vi "Sony LANC remote.vi"() -> ()   [LabVIEW 2023]
panel:
  in  "plus":bool
  in  "minus":bool
  in  "15key":bool
  in  "16key":bool
  in  "7key":bool
  in  "8key":bool
  in  "9key":bool
  in  "10key":bool
  in  "11key":bool
  in  "12key":bool
  in  "13key":bool
  in  "14key":bool
  in  "1key":bool caption="Keypad"
  in  "2key":bool
  in  "3key":bool
  in  "4key":bool
  in  "5key":bool
  in  "6key":bool
  in  "EEPROM_store":bool
  in  "EEPROM_read":bool
  in  "valup":bool caption="Data"
  in  "valdn":bool
  in  "adup":bool caption="Addr"
  in  "addn":bool
  in  "pgup":bool caption="Page"
  in  "pgdn":bool
  out "EEPROM":string
  in  "send_custom":bool
  in  "eject":bool
  in  "fwd":bool
  in  "rew":bool
  in  "stop":bool
  in  "pause":bool
  in  "play":bool
  in  "enter":bool
  in  "menu":bool
  in  "right":bool
  in  "left":bool
  in  "up":bool
  in  "down":bool
  in  "Command":string(combo)
  out "Time":string
  out "Date":string
  out "data_code":cluster{"year/hour":u32, "month/min":u32}
  out "data_type":u8(ring) items=["Undefined"=0, "Date"=3, "Time"=4]
  out "Remaining time":string
  out "Real time counter":string
  out "RCTC":bool
  out "min_sec":cluster{"min":u32, "sec":u32}
  out "Decimal counter":u32
  out "Features":T1 {"Capability" items=["V8"=0, "DV"=1, "DV"=2, "Hi8"=4]; "Input" items=["Tuner"=0, "Sim."=1, "Line"=3]; "Thickness" items=["10µm", "13µm"]; "Type" items=["MP", "ME"]; "Speed" items=["SP", "LP"]}
  out "Status":string
  out "EOP":bool
  in  "stop":bool
  in  "send":bool
  in  "cmd":string caption="Custom cmd (2 bytes hex)"
  # "Tape"
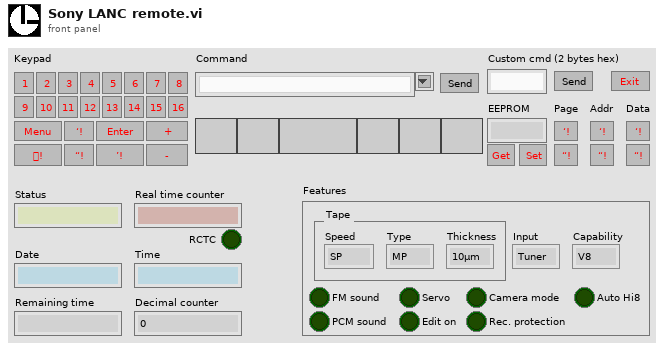
[diagram p1: front panel]
types:
  T1 = cluster{"Speed":u8, "FM sound":bool, "PCM sound":bool, "Camera mode":bool, "Rec. protection":bool, "Type":u8, "Thickness":u8, "Servo":bool, "Input":u8, "Capability":u8, "Edit on":bool, "Auto Hi8":bool}
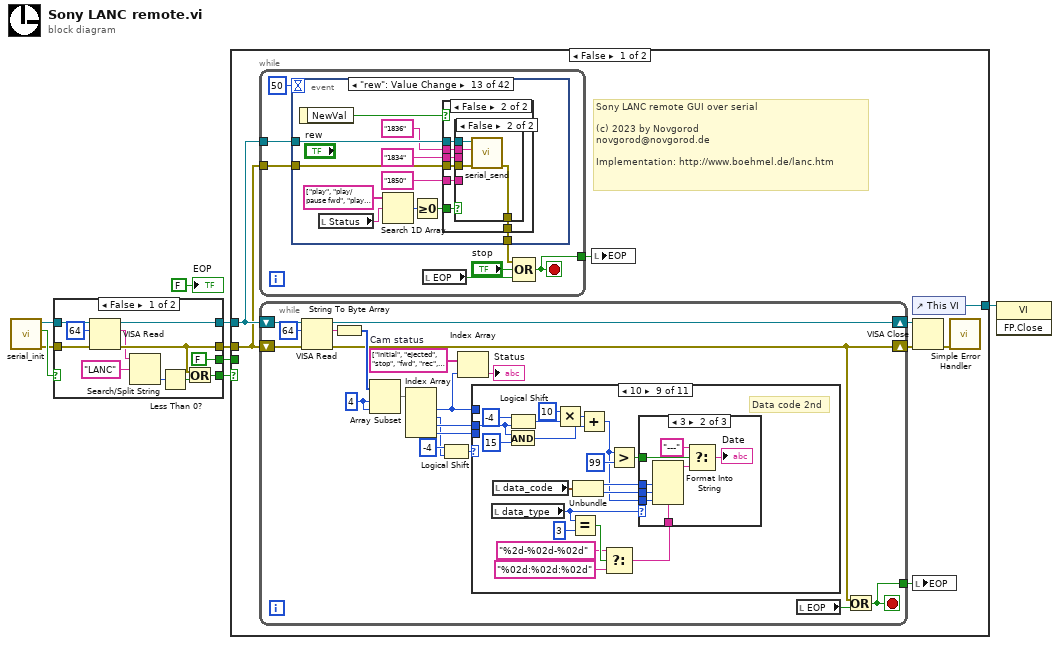
[diagram p0: block diagram]
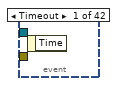
[diagram p3: hidden frame]
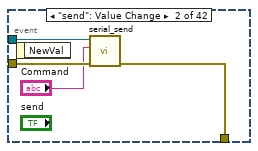
[diagram p4: hidden frame]
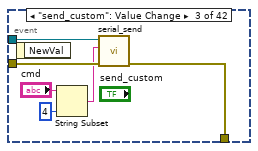
[diagram p5: hidden frame]
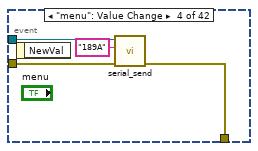
[diagram p6: hidden frame]
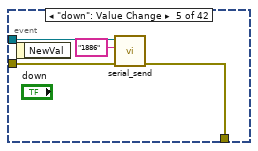
[diagram p7: hidden frame]
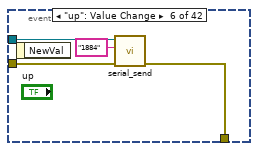
[diagram p8: hidden frame]
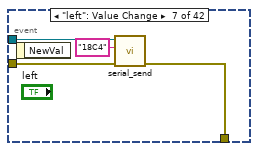
[diagram p9: hidden frame]
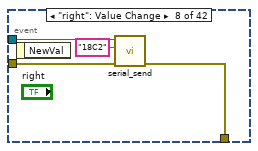
[diagram p10: hidden frame]
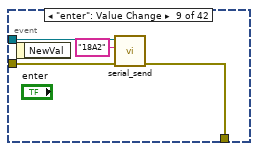
[diagram p11: hidden frame]
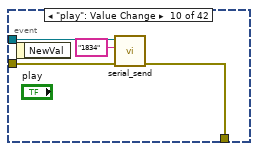
[diagram p12: hidden frame]
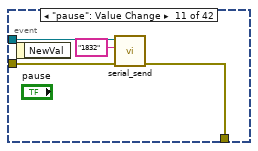
[diagram p13: hidden frame]
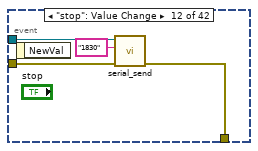
[diagram p14: hidden frame]
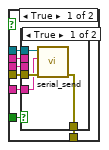
[diagram p15: hidden frame]
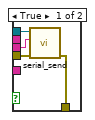
[diagram p17: hidden frame]
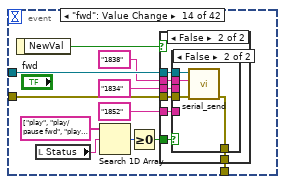
[diagram p18: hidden frame]
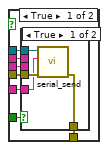
[diagram p19: hidden frame]
diagram:
  n1 = call "serial_init.vi"() -> ("error out"=w3:errorcluster, "Cancelled?"=w4:bool, "VISA out"=w5:refnum<visa-resource-name>)  [unwired: 9 in]
  n2 = case shown="False" w4 {
    selector: w4 -> [_ w21]
    tunnel: [w20 w22] -> w9
    tunnel: [w19 _] -> w8
    tunnel: [w18 w21] -> w7
    tunnel: w5 -> [w12 w22]
    tunnel: w3 -> [w11 _]
    tunnel: [FALSE w21] -> w1
    frame False {
      n3 = VISA Read(VISA resource name=w12, byte count=u32 64, error in (no error)=w11) -> (VISA resource name out=w20:refnum<visa-resource-name>, read buffer=w16:string, error out=w19:errorcluster)  [unwired: 1 out]
      n4 = Search/Split String(string=w16, search string/char (-)="LANC") -> (offset of match=w14:i32)  [unwired: 1 in, 2 out]
      n5 = Less Than 0?(x=w14) -> (x < 0?=w13:bool)
      n6 = Or(x=w19, y=w13) -> (x .or. y?=w18:bool)
    }
    frame True {
    }
  }
  n7 = case shown="False" w7 {
    tunnel: w9 -> [w27 w470]
    tunnel: w8 -> [w26 _]
    tunnel: [w23 w471] -> w2
    tunnel: w1 -> [_ w469]
    frame False {
      # "Sony LANC remote GUI over serial\n\n(c) 2023 by Novgorod\nnovgorod@novgorod.de\n\nImplementation: http://www.boehmel.de/lanc.htm"
      n8 = while {
        tunnel: w26 -> [w35]
        tunnel: w27 -> [w36]
        tunnel: [w32] -> w24
        stop <- w32 stop-if-true
        n9 = event shown="[12] \"rew\": Value Change" {
          selector: _ -> [_ _ _ _ _ _ _ _ _ _ _ _ _ _ _ _ _ _ _ _ _ _ _ _ _ _ _ _ _ _ _ _ _ _ _ _ _ _ _ _ _ _]
          dyn-events: _ -> [_ _ _ _ _ _ _ _ _ _ _ _ _ _ _ _ _ _ _ _ _ _ _ _ _ _ _ _ _ _ _ _ _ _ _ _ _ _ _ _ _ _]
          timeout: 50 -> [_ _ _ _ _ _ _ _ _ _ _ _ _ _ _ _ _ _ _ _ _ _ _ _ _ _ _ _ _ _ _ _ _ _ _ _ _ _ _ _ _ _]
          tunnel: w36 -> [_ w41 w47 w51 w55 w59 w63 w67 w71 w75 w79 w83 w94 w132 w163 w167 w171 w175 w179 w183 w187 w191 w195 w199 w203 w207 w211 w215 w219 w223 w227 w231 w236 w245 w249 w253 w257 w261 w265 w269 w273 _]
          tunnel: w35 -> [_ w40 w46 w50 w54 w58 w62 w66 w70 w74 w78 w82 w93 w131 w162 w166 w170 w174 w178 w182 w186 w190 w194 w198 w202 w206 w210 w214 w218 w222 w226 w230 w235 w244 w248 w252 w256 w260 w264 w268 w272 _]
          tunnel: [_ w39 w45 w49 w53 w57 w61 w65 w69 w73 w77 w81 w92 w130 w161 w165 w169 w173 w177 w181 w185 w189 w193 w197 w201 w205 w209 w213 w217 w221 w225 w229 w234 w243 w247 w251 w255 w259 w263 w267 w271 errorcluster {"status"=TRUE, "code"=0, "source"=""} ("error out")] -> w34
          event Timeout {
            n10 = event-data() -> ()  [unwired: 1 in, 1 out]
          }
          event "send": Value Change {
            n11 = event-data() -> ()  [unwired: 1 in, 1 out]
            n12 = call "serial_send.vi"("error in (no error)"=w40, "Send buffer"="Command", "VISA in"=w41) -> ("error out"=w39:errorcluster)  [unwired: 7 in, 1 out]
          }
          event "send_custom": Value Change {
            n13 = event-data() -> ()  [unwired: 1 in, 1 out]
            n14 = String Subset(string="cmd", length (rest)=4 ("length (rest)")) -> (substring=w42:string)  [unwired: 1 in]
            n15 = call "serial_send.vi"("error in (no error)"=w46, "Send buffer"=w42, "VISA in"=w47) -> ("error out"=w45:errorcluster)  [unwired: 7 in, 1 out]
          }
          event "menu": Value Change {
            n16 = event-data() -> ()  [unwired: 1 in, 1 out]
            n17 = call "serial_send.vi"("error in (no error)"=w50, "Send buffer"="189A", "VISA in"=w51) -> ("error out"=w49:errorcluster)  [unwired: 7 in, 1 out]
          }
          event "down": Value Change {
            n18 = event-data() -> ()  [unwired: 1 in, 1 out]
            n19 = call "serial_send.vi"("error in (no error)"=w54, "Send buffer"="1886", "VISA in"=w55) -> ("error out"=w53:errorcluster)  [unwired: 7 in, 1 out]
          }
          event "up": Value Change {
            n20 = event-data() -> ()  [unwired: 1 in, 1 out]
            n21 = call "serial_send.vi"("error in (no error)"=w58, "Send buffer"="1884", "VISA in"=w59) -> ("error out"=w57:errorcluster)  [unwired: 7 in, 1 out]
          }
          event "left": Value Change {
            n22 = event-data() -> ()  [unwired: 1 in, 1 out]
            n23 = call "serial_send.vi"("error in (no error)"=w62, "Send buffer"="18C4", "VISA in"=w63) -> ("error out"=w61:errorcluster)  [unwired: 7 in, 1 out]
          }
          event "right": Value Change {
            n24 = event-data() -> ()  [unwired: 1 in, 1 out]
            n25 = call "serial_send.vi"("error in (no error)"=w66, "Send buffer"="18C2", "VISA in"=w67) -> ("error out"=w65:errorcluster)  [unwired: 7 in, 1 out]
          }
          event "enter": Value Change {
            n26 = event-data() -> ()  [unwired: 1 in, 1 out]
            n27 = call "serial_send.vi"("error in (no error)"=w70, "Send buffer"="18A2", "VISA in"=w71) -> ("error out"=w69:errorcluster)  [unwired: 7 in, 1 out]
          }
          event "play": Value Change {
            n28 = event-data() -> ()  [unwired: 1 in, 1 out]
            n29 = call "serial_send.vi"("error in (no error)"=w74, "Send buffer"="1834", "VISA in"=w75) -> ("error out"=w73:errorcluster)  [unwired: 7 in, 1 out]
          }
          event "pause": Value Change {
            n30 = event-data() -> ()  [unwired: 1 in, 1 out]
            n31 = call "serial_send.vi"("error in (no error)"=w78, "Send buffer"="1832", "VISA in"=w79) -> ("error out"=w77:errorcluster)  [unwired: 7 in, 1 out]
          }
          event "stop": Value Change {
            n32 = event-data() -> ()  [unwired: 1 in, 1 out]
            n33 = call "serial_send.vi"("error in (no error)"=w82, "Send buffer"="1830", "VISA in"=w83) -> ("error out"=w81:errorcluster)  [unwired: 7 in, 1 out]
          }
          event "rew": Value Change {
            n34 = event-data() -> ("NewVal"=w87:bool)  [unwired: 1 in]
            n35 = local read "Status"() -> (w89:string)
            n36 = Search 1D Array(1D array=string[] ["play", "play/pause fwd", "play/pause rev", "cue", "rev", "x1 fwd", "1/5 fwd", "x1 rev", "1/5 rev", "1/10 fwd", "1/10 rev", "x2/x3 fwd", "x2/x3 rev", "x9 fwd", "x9 rev", "edit-s rev", "frame sea. rev", "x14 fwd", "x14 rev", "edit search+", "edit search-", "edit-s fwd", "frame sea. cue"], element=w89) -> (index of element=w90:i32)  [unwired: 1 in]
            n37 = Greater Or Equal To 0?(x=w90) -> (x >= 0?=w88:bool)
            n38 = case shown="False" w87 {
              tunnel: w94 -> [w101 w113]
              tunnel: w93 -> [w100 w112]
              tunnel: [w99 w111] -> w92
              tunnel: "1836" -> [w98 w110]
              tunnel: w88 -> [w97 w109]
              tunnel: "1850" -> [w96 w108]
              tunnel: "1834" -> [w95 w107]
              frame True {
                n39 = case shown="True" w97 {
                  tunnel: w101 -> [w105 _]
                  tunnel: w100 -> [w104 w106]
                  tunnel: [w103 w106] -> w99
                  tunnel: w98 -> [_ _]
                  tunnel: w96 -> [w102 _]
                  tunnel: w95 -> [_ _]
                  frame True {
                    n40 = call "serial_send.vi"("error in (no error)"=w104, "Send buffer"=w102, "VISA in"=w105) -> ("error out"=w103:errorcluster)  [unwired: 7 in, 1 out]
                  }
                  frame False {
                  }
                }
              }
              frame False {
                n41 = case shown="False" w109 {
                  tunnel: w113 -> [w117 w119]
                  tunnel: w112 -> [w116 w121]
                  tunnel: [w115 w118] -> w111
                  tunnel: w110 -> [_ w120]
                  tunnel: w108 -> [_ _]
                  tunnel: w107 -> [w114 _]
                  frame True {
                    n42 = call "serial_send.vi"("error in (no error)"=w116, "Send buffer"=w114, "VISA in"=w117) -> ("error out"=w115:errorcluster)  [unwired: 7 in, 1 out]
                  }
                  frame False {
                    n43 = call "serial_send.vi"("error in (no error)"=w121, "Send buffer"=w120, "VISA in"=w119) -> ("error out"=w118:errorcluster)  [unwired: 7 in, 1 out]
                  }
                }
              }
            }
          }
          event "fwd": Value Change {
            n44 = event-data() -> ("NewVal"=w125:bool)  [unwired: 1 in]
            n45 = local read "Status"() -> (w127:string)
            n46 = Search 1D Array(1D array=string[] ["play", "play/pause fwd", "play/pause rev", "cue", "rev", "x1 fwd", "1/5 fwd", "x1 rev", "1/5 rev", "1/10 fwd", "1/10 rev", "x2/x3 fwd", "x2/x3 rev", "x9 fwd", "x9 rev", "edit-s rev", "frame sea. rev", "x14 fwd", "x14 rev", "edit search+", "edit search-", "edit-s fwd", "frame sea. cue"], element=w127) -> (index of element=w128:i32)  [unwired: 1 in]
            n47 = Greater Or Equal To 0?(x=w128) -> (x >= 0?=w126:bool)
            n48 = case shown="False" w125 {
              tunnel: w132 -> [w139 w151]
              tunnel: w131 -> [w138 w150]
              tunnel: [w137 w149] -> w130
              tunnel: "1838" -> [w136 w148]
              tunnel: w126 -> [w135 w147]
              tunnel: "1852" -> [w134 w146]
              tunnel: "1834" -> [w133 w145]
              frame True {
                n49 = case shown="True" w135 {
                  tunnel: w139 -> [w143 _]
                  tunnel: w138 -> [w142 w144]
                  tunnel: [w141 w144] -> w137
                  tunnel: w136 -> [_ _]
                  tunnel: w134 -> [w140 _]
                  tunnel: w133 -> [_ _]
                  frame True {
                    n50 = call "serial_send.vi"("error in (no error)"=w142, "Send buffer"=w140, "VISA in"=w143) -> ("error out"=w141:errorcluster)  [unwired: 7 in, 1 out]
                  }
                  frame False {
                  }
                }
              }
              frame False {
                n51 = case shown="False" w147 {
                  tunnel: w151 -> [w155 w158]
                  tunnel: w150 -> [w154 w159]
                  tunnel: [w153 w156] -> w149
                  tunnel: w148 -> [_ w157]
                  tunnel: w146 -> [_ _]
                  tunnel: w145 -> [w152 _]
                  frame True {
                    n52 = call "serial_send.vi"("error in (no error)"=w154, "Send buffer"=w152, "VISA in"=w155) -> ("error out"=w153:errorcluster)  [unwired: 7 in, 1 out]
                  }
                  frame False {
                    n53 = call "serial_send.vi"("error in (no error)"=w159, "Send buffer"=w157, "VISA in"=w158) -> ("error out"=w156:errorcluster)  [unwired: 7 in, 1 out]
                  }
                }
              }
            }
          }
          event "1key": Value Change {
            n54 = event-data() -> ()  [unwired: 1 in, 1 out]
            n55 = call "serial_send.vi"("error in (no error)"=w162, "Send buffer"="1800", "VISA in"=w163) -> ("error out"=w161:errorcluster)  [unwired: 7 in, 1 out]
          }
          event "2key": Value Change {
            n56 = event-data() -> ()  [unwired: 1 in, 1 out]
            n57 = call "serial_send.vi"("error in (no error)"=w166, "Send buffer"="1802", "VISA in"=w167) -> ("error out"=w165:errorcluster)  [unwired: 7 in, 1 out]
          }
          event "3key": Value Change {
            n58 = event-data() -> ()  [unwired: 1 in, 1 out]
            n59 = call "serial_send.vi"("error in (no error)"=w170, "Send buffer"="1804", "VISA in"=w171) -> ("error out"=w169:errorcluster)  [unwired: 7 in, 1 out]
          }
          event "4key": Value Change {
            n60 = event-data() -> ()  [unwired: 1 in, 1 out]
            n61 = call "serial_send.vi"("error in (no error)"=w174, "Send buffer"="1806", "VISA in"=w175) -> ("error out"=w173:errorcluster)  [unwired: 7 in, 1 out]
          }
          event "5key": Value Change {
            n62 = event-data() -> ()  [unwired: 1 in, 1 out]
            n63 = call "serial_send.vi"("error in (no error)"=w178, "Send buffer"="1808", "VISA in"=w179) -> ("error out"=w177:errorcluster)  [unwired: 7 in, 1 out]
          }
          event "6key": Value Change {
            n64 = event-data() -> ()  [unwired: 1 in, 1 out]
            n65 = call "serial_send.vi"("error in (no error)"=w182, "Send buffer"="180A", "VISA in"=w183) -> ("error out"=w181:errorcluster)  [unwired: 7 in, 1 out]
          }
          event "7key": Value Change {
            n66 = event-data() -> ()  [unwired: 1 in, 1 out]
            n67 = call "serial_send.vi"("error in (no error)"=w186, "Send buffer"="180C", "VISA in"=w187) -> ("error out"=w185:errorcluster)  [unwired: 7 in, 1 out]
          }
          event "8key": Value Change {
            n68 = event-data() -> ()  [unwired: 1 in, 1 out]
            n69 = call "serial_send.vi"("error in (no error)"=w190, "Send buffer"="180E", "VISA in"=w191) -> ("error out"=w189:errorcluster)  [unwired: 7 in, 1 out]
          }
          event "9key": Value Change {
            n70 = event-data() -> ()  [unwired: 1 in, 1 out]
            n71 = call "serial_send.vi"("error in (no error)"=w194, "Send buffer"="1810", "VISA in"=w195) -> ("error out"=w193:errorcluster)  [unwired: 7 in, 1 out]
          }
          event "10key": Value Change {
            n72 = event-data() -> ()  [unwired: 1 in, 1 out]
            n73 = call "serial_send.vi"("error in (no error)"=w198, "Send buffer"="1812", "VISA in"=w199) -> ("error out"=w197:errorcluster)  [unwired: 7 in, 1 out]
          }
          event "11key": Value Change {
            n74 = event-data() -> ()  [unwired: 1 in, 1 out]
            n75 = call "serial_send.vi"("error in (no error)"=w202, "Send buffer"="1814", "VISA in"=w203) -> ("error out"=w201:errorcluster)  [unwired: 7 in, 1 out]
          }
          event "12key": Value Change {
            n76 = event-data() -> ()  [unwired: 1 in, 1 out]
            n77 = call "serial_send.vi"("error in (no error)"=w206, "Send buffer"="1816", "VISA in"=w207) -> ("error out"=w205:errorcluster)  [unwired: 7 in, 1 out]
          }
          event "13key": Value Change {
            n78 = event-data() -> ()  [unwired: 1 in, 1 out]
            n79 = call "serial_send.vi"("error in (no error)"=w210, "Send buffer"="1818", "VISA in"=w211) -> ("error out"=w209:errorcluster)  [unwired: 7 in, 1 out]
          }
          event "14key": Value Change {
            n80 = event-data() -> ()  [unwired: 1 in, 1 out]
            n81 = call "serial_send.vi"("error in (no error)"=w214, "Send buffer"="181A", "VISA in"=w215) -> ("error out"=w213:errorcluster)  [unwired: 7 in, 1 out]
          }
          event "15key": Value Change {
            n82 = event-data() -> ()  [unwired: 1 in, 1 out]
            n83 = call "serial_send.vi"("error in (no error)"=w218, "Send buffer"="181C", "VISA in"=w219) -> ("error out"=w217:errorcluster)  [unwired: 7 in, 1 out]
          }
          event "16key": Value Change {
            n84 = event-data() -> ()  [unwired: 1 in, 1 out]
            n85 = call "serial_send.vi"("error in (no error)"=w222, "Send buffer"="181E", "VISA in"=w223) -> ("error out"=w221:errorcluster)  [unwired: 7 in, 1 out]
          }
          event "plus": Value Change {
            n86 = event-data() -> ()  [unwired: 1 in, 1 out]
            n87 = call "serial_send.vi"("error in (no error)"=w226, "Send buffer"="1820", "VISA in"=w227) -> ("error out"=w225:errorcluster)  [unwired: 7 in, 1 out]
          }
          event "minus": Value Change {
            n88 = event-data() -> ()  [unwired: 1 in, 1 out]
            n89 = call "serial_send.vi"("error in (no error)"=w230, "Send buffer"="1822", "VISA in"=w231) -> ("error out"=w229:errorcluster)  [unwired: 7 in, 1 out]
          }
          event "eject": Value Change {
            n90 = event-data() -> ()  [unwired: 1 in, 1 out]
            n91 = Two Button Dialog(message="Eject tape?") -> (T button?=w232:bool)  [unwired: 2 in]
            n92 = case shown="True" w232 {
              tunnel: w236 -> [_ w241]
              tunnel: w235 -> [w237 w240]
              tunnel: [w237 w239] -> w234
              frame False {
              }
              frame True {
                n93 = call "serial_send.vi"("error in (no error)"=w240, "Send buffer"="182C", "VISA in"=w241) -> ("error out"=w239:errorcluster)  [unwired: 7 in, 1 out]
              }
            }
          }
          event "EEPROM_read": Value Change {
            n94 = event-data() -> ()  [unwired: 1 in, 1 out]
            n95 = call "serial_send.vi"("error in (no error)"=w244, "Send buffer"="FF00", "VISA in"=w245) -> ("error out"=w243:errorcluster)  [unwired: 7 in, 1 out]
          }
          event "EEPROM_store": Value Change {
            n96 = event-data() -> ()  [unwired: 1 in, 1 out]
            n97 = call "serial_send.vi"("error in (no error)"=w248, "Send buffer"="FF32", "VISA in"=w249) -> ("error out"=w247:errorcluster)  [unwired: 7 in, 1 out]
          }
          event "pgup": Value Change {
            n98 = event-data() -> ()  [unwired: 1 in, 1 out]
            n99 = call "serial_send.vi"("error in (no error)"=w252, "Send buffer"="FF67", "VISA in"=w253) -> ("error out"=w251:errorcluster)  [unwired: 7 in, 1 out]
          }
          event "pgdn": Value Change {
            n100 = event-data() -> ()  [unwired: 1 in, 1 out]
            n101 = call "serial_send.vi"("error in (no error)"=w256, "Send buffer"="FF65", "VISA in"=w257) -> ("error out"=w255:errorcluster)  [unwired: 7 in, 1 out]
          }
          event "adup": Value Change {
            n102 = event-data() -> ()  [unwired: 1 in, 1 out]
            n103 = call "serial_send.vi"("error in (no error)"=w260, "Send buffer"="FF38", "VISA in"=w261) -> ("error out"=w259:errorcluster)  [unwired: 7 in, 1 out]
          }
          event "addn": Value Change {
            n104 = event-data() -> ()  [unwired: 1 in, 1 out]
            n105 = call "serial_send.vi"("error in (no error)"=w264, "Send buffer"="FF36", "VISA in"=w265) -> ("error out"=w263:errorcluster)  [unwired: 7 in, 1 out]
          }
          event "valup": Value Change {
            n106 = event-data() -> ()  [unwired: 1 in, 1 out]
            n107 = call "serial_send.vi"("error in (no error)"=w268, "Send buffer"="FF34", "VISA in"=w269) -> ("error out"=w267:errorcluster)  [unwired: 7 in, 1 out]
          }
          event "valdn": Value Change {
            n108 = event-data() -> ()  [unwired: 1 in, 1 out]
            n109 = call "serial_send.vi"("error in (no error)"=w272, "Send buffer"="FF30", "VISA in"=w273) -> ("error out"=w271:errorcluster)  [unwired: 7 in, 1 out]
          }
          event Panel Close? {
            n110 = event-data() -> ()  [unwired: 1 in, 1 out]
            n111 = event-data("Discard?"=TRUE) -> ()  [unwired: 1 in, 1 out]
          }
        }
        n112 = local read "EOP"() -> (w31:bool)
        n113 = Compound Arithmetic op=OR(w34, "stop", w31) -> (w32:bool)
      }
      n114 = while {
        shift-right: [w292] -> w29
        shift-left: w27 -> [w294]
        shift-right: [w287] -> w30
        shift-left: w26 -> [w293]
        tunnel: [w276] -> w25
        stop <- w276 stop-if-true
        w284 = string[] ["initial", "ejected", "stop", "fwd", "rec", "", "play", "play/pause fwd", "AL insert", "", "", "", "", "", "", "page 0", "", "dew cass. out", "laod", "", "rec/pause", "", "", "frame fwd", "AL ins-pause", "", "", "", "", "", "", "page 1", "", "ejecting", "cassette busy", "", "timer-rec", "", "x1 fwd", "1/5 fwd", "AR insert", "", "", "", "", "", "", "page 2", "", "unload", "low-battery", "go zero/play f.", "timer-rec s.", "", "x1 rev", "1/5 rev", "AR ins-pause", "", "", "", "", "", "", "page 3", "", "", "dew stop", "fwd mem stop", "AV insert", "", "cue", "1/10 fwd", "AL+V insert", "", "", "", "", "", "", "page 4", "", "", "emergency", "", "AV ins.-pause", "", "rev", "1/10 rev", "AL+V ins-ps", "", "", "", "", "", "", "page 5", "", "", "tape end", "", "video insert", "", "x2/x3 fwd", "frame fwd", "AR+V insert", "", "", "", "", "", "", "page 6", "", "", "tape top", "", "video ins.-ps", "", "x2/x3 rev", "frame rev", "AL+R ins-ps", "", "", "", "", "", "", "page 7", "", "", "", "rew", "audio dub", "edit search+", "x9 fwd", "", "", "", "", "", "", "", "", "page 8", "", "", "stp after zero", "", "a. dub pause", "edit search-", "x9 rev", "play/pause rev", "", "", "", "", "", "", "", "page 9", "", "", "load emer.", "auto-play", "cam rec", "edit-s fwd", "frame sea. cue", "", "", "", "", "", "", "", "", "page A", "", "unload emerg.", "stop emerg. 1", "go zero/play r.", "cam stby", "edit-s rev", "frame sea. rev", "", "", "", "", "", "", "", "", "page B", "", "", "stop emerg. 2", "rew mem stop", "", "", "x14 fwd", "", "", "", "", "", "", "", "", "page C", "", "", "", "hi-speed rew", "", "", "x14 rev", "", "", "", "", "", "", "", "", "page D", "", "", "stop NC", "", "", "", "", "", "", "", "", "", "", "", "", "page E", "", "", "", "", "", "edit pause", "", "", "", "", "", "", "", "", "", "page F"]  # Cam status
        w286 = 4 ("index")
        n115 = VISA Read(VISA resource name=w294, byte count=u32 64, error in (no error)=w293) -> (VISA resource name out=w292:refnum<visa-resource-name>, read buffer=w290:string, error out=w287:errorcluster)  [unwired: 1 out]
        n116 = String To Byte Array(string=w290) -> (unsigned byte array=w289:u8[])
        n117 = Array Subset(array=w289, index=w286, length=w286) -> (w285:u8[])
        n118 = Index Array(array=w285) -> (element #1=w277:u8, element #2=w278:u8, element #3=w279:u8, element #4=w280:u8)  [unwired: 4 in]
        n119 = Logical Shift(y=i16 -4, x=w278) -> (x << y=w281:u8)
        n120 = Index Array(array=w284, index=w277) -> (element=→"Status":string)
        n121 = case shown="10" w281 {
          tunnel: w280 -> [_ w317 w330 w347 w374 w396 w399 w411 _ w456 w463]
          tunnel: w279 -> [_ w318 w331 w348 w382 w397 _ w412 w433 w460 w464]
          tunnel: w277 -> [_ _ _ _ _ _ _ _ _ _ w468]
          frame 0, Default {
          }
          frame 1 {
            # "Status V8 and Hi8"
            n122 = Join Numbers(hi=w317, lo=w318) -> ((hi.lo)=w316:u16)
            n123 = Number To Boolean Array(number=w316) -> (Boolean array=w315:bool[])
            n124 = Index Array(array=w315, index #2=2 ("index"), index #8=11 ("index"), index #10=14 ("index")) -> (element #1=w314:bool, element #2=w303:bool, element #3=w302:bool, element #4=w301:bool, element #5=w300:bool, element #6=w312:bool, element #7=w311:bool, element #8=w297:bool, element #9=w309:bool, element #10=w307:bool)  [unwired: 7 in]
            n125 = Boolean To (0,1)(Boolean=w314) -> (0, 1=w304:i16)
            n126 = Boolean To (0,1)(Boolean=w312) -> (0, 1=w299:i16)
            n127 = Boolean To (0,1)(Boolean=w311) -> (0, 1=w298:i16)
            n128 = Build Array(w309, w307) -> (w306:bool[])
            n129 = local read "Features"() -> (w305:T1)
            n130 = Boolean Array To Number(Boolean array=w306) -> (number=w296:u32)
            n131 = Bundle(cluster=w305, "Speed"=w304, "FM sound"=w303, "PCM sound"=w302, "Camera mode"=w301, "Rec. protection"=w300, "Type"=w299, "Thickness"=w298, "Servo"=w297, "Input"=w296) -> (→"Features":T1)  [unwired: 3 in]
          }
          frame 2 {
            # "Decimal counter"
            n132 = Logical Shift(y=i16 -4, x=w330) -> (x << y=w326:u8)
            n133 = And(x=w330, y=u8 15) -> (x .and. y?=w324:u8)
            n134 = Logical Shift(y=i16 -4, x=w331) -> (x << y=w329:u8)
            n135 = And(x=w331, y=u8 15) -> (x .and. y?=w322:u8)
            n136 = Multiply(x=u32 10, y=w329) -> (x*y=w323:u32)
            n137 = Multiply(x=u32 1000, y=w326) -> (x*y=w321:u32)
            n138 = Multiply(x=u32 100, y=w324) -> (x*y=w320:u32)
            n139 = Compound Arithmetic op=ADD(w323, w322, w321, w320) -> (→"Decimal counter":u32)
          }
          frame 3 {
            # "Real time counter 1st"
            n140 = Logical Shift(y=i16 -4, x=w347) -> (x << y=w343:u8)
            n141 = And(x=w347, y=u8 15) -> (x .and. y?=w339:u8)
            n142 = Logical Shift(y=i16 -4, x=w348) -> (x << y=w346:u8)
            n143 = And(x=w348, y=u8 15) -> (x .and. y?=w341:u8)
            n144 = Multiply(x=u32 10, y=w346) -> (x*y=w342:u32)
            n145 = Multiply(x=u32 10, y=w343) -> (x*y=w340:u32)
            n146 = Add(x=w342, y=w341) -> (x+y=w337:u32)
            n147 = Add(x=w340, y=w339) -> (x+y=w338:u32)
            n148 = Bundle(w338, w337) -> (→"min_sec":cluster{u32, u32})  [unwired: 1 in]
          }
          frame 4 {
            # "Real time counter 2nd"
            n149 = Number To Boolean Array(number=w374) -> (Boolean array=w373:bool[])
            n150 = Logical Shift(y=i16 -4, x=w374) -> (x << y=w361:u8)
            n151 = And(x=w374, y=u8 15) -> (x .and. y?=w375:u8)
            n152 = Logical Shift(y=i16 -4, x=w382) -> (x << y=w381:u8)
            n153 = And(x=w382, y=u8 15) -> (x .and. y?=w377:u8)
            n154 = Index Array(array=w373, index #1=6 ("index")) -> (element #1=→"RCTC":bool, element #2=w370:bool)  [unwired: 1 in]
            n155 = local read "min_sec"() -> (w364:cluster{"min":u32, "sec":u32})
            n156 = And(x=u8 3, y=w361) -> (x .and. y?=w359:u8)
            n157 = Multiply(x=u32 10, y=w381) -> (x*y=w378:u32)
            n158 = Add(x=w378, y=w377) -> (x+y=w358:u32)
            n159 = Multiply(x=u32 10, y=w359) -> (x*y=w376:u32)
            n160 = Select(t="-", s=w370, f="") -> (s? t:f=w367:string)
            n161 = Unbundle(w364) -> ("min"=w363:u32, "sec"=w362:u32)
            n162 = Add(x=w376, y=w375) -> (x+y=w365:u32)
            n163 = Greater?(x=w358, y=u32 99) -> (0:w356:bool)
            n164 = Format Into String(format string="%d:%02d:%02d:%02d", initial string=w367, w358, w363, w362, w365) -> (resulting string=w355:string)  [unwired: 1 in, 1 out]
            n165 = Select(t="---", s=w356, f=w355) -> (s? t:f=→"Real time counter":string)
          }
          frame 5 {
            w388 = u8 15
            # "Remaining time"
            n166 = Logical Shift(y=i16 -4, x=w397) -> (x << y=w395:u8)
            n167 = And(x=w397, y=w388) -> (x .and. y?=w392:u8)
            n168 = And(x=w396, y=w388) -> (x .and. y?=w389:u8)
            n169 = Multiply(x=u32 10, y=w395) -> (x*y=w393:u32)
            n170 = Add(x=w393, y=w392) -> (x+y=w390:u32)
            n171 = Format Into String(format string="%d:%02d", w389, w390) -> (resulting string=→"Remaining time":string)  [unwired: 2 in, 1 out]
          }
          frame 8 {
            # "Data code type"
            "data_type" <- w399
          }
          frame 9 {
            # "Data code 1st"
            n172 = Logical Shift(y=i16 -4, x=w411) -> (x << y=w407:u8)
            n173 = And(x=w411, y=u8 15) -> (x .and. y?=w403:u8)
            n174 = Logical Shift(y=i16 -4, x=w412) -> (x << y=w410:u8)
            n175 = And(x=w412, y=u8 15) -> (x .and. y?=w405:u8)
            n176 = Multiply(x=u32 10, y=w410) -> (x*y=w406:u32)
            n177 = Multiply(x=u32 10, y=w407) -> (x*y=w404:u32)
            n178 = Add(x=w406, y=w405) -> (x+y=w401:u32)
            n179 = Add(x=w404, y=w403) -> (x+y=w402:u32)
            n180 = Bundle(w401, w402) -> (→"data_code":cluster{u32, u32})  [unwired: 1 in]
          }
          frame 10 {
            # "Data code 2nd"
            n181 = local read "data_type"() -> (w425:u8)
            n182 = local read "data_code"() -> (w428:cluster{"year/hour":u32, "month/min":u32})
            n183 = Logical Shift(y=i16 -4, x=w433) -> (x << y=w432:u8)
            n184 = And(x=w433, y=u8 15) -> (x .and. y?=w429:u8)
            n185 = Multiply(x=u32 10, y=w432) -> (x*y=w430:u32)
            n186 = Equal?(x=w425, y=u8 3) -> (x = y?=w424:bool)
            n187 = Unbundle(w428) -> ("year/hour"=w427:u32, "month/min"=w426:u32)
            n188 = Add(x=w430, y=w429) -> (x+y=w418:u32)
            n189 = Select(t="%2d-%02d-%02d" ("format string"), s=w424, f="%02d:%02d:%02d" ("format string")) -> (s? t:f=w421:string)
            n190 = Greater?(x=w418, y=u32 99) -> (0:w417:bool)
            n191 = case shown="3" w425 {
              tunnel: w421 -> [_ w443 w451]
              tunnel: w418 -> [_ w442 w450]
              tunnel: w427 -> [_ w441 w449]
              tunnel: w426 -> [_ w440 w448]
              tunnel: w417 -> [_ w437 w446]
              frame 0, Default {
              }
              frame 3 {
                n192 = Format Into String(format string=w443, w441, w440, w442) -> (resulting string=w438:string)  [unwired: 2 in, 1 out]
                n193 = Select(t="---", s=w437, f=w438) -> (s? t:f=→"Date":string)
              }
              frame 4 {
                n194 = Format Into String(format string=w451, w449, w448, w450) -> (resulting string=w445:string)  [unwired: 2 in, 1 out]
                n195 = Select(t="---", s=w446, f=w445) -> (s? t:f=→"Time":string)
              }
            }
          }
          frame 12 {
            # "Status Hi8, DV"
            n196 = Number To Boolean Array(number=w456) -> (Boolean array=w455:bool[])
            n197 = And(x=w460, y=u8 15) -> (x .and. y?=w458:u8)
            n198 = Index Array(array=w455, index #1=2 ("index")) -> (element #1=w453:bool, element #2=w452:bool)  [unwired: 1 in]
            n199 = local read "Features"() -> (w459:T1)
            n200 = Bundle By Name(cluster=w459, "Capability"=w458, "Edit on"=w453, "Auto Hi8"=w452) -> (w457:T1)
            n201 = local write "Features"(w457) -> ()
          }
          frame 15 {
            # "EEPROM"
            n202 = Logical Shift(y=i16 -4, x=w468) -> (x << y=w465:u8)
            n203 = Format Into String(format string="%x:%02x:%02x", w465, w464, w463) -> (resulting string=→"EEPROM":string)  [unwired: 2 in, 1 out]
          }
        }
        n204 = local read "EOP"() -> (w288:bool)
        n205 = Or(x=w287, y=w288) -> (x .or. y?=w276:bool)
      }
      n206 = local write "EOP"(w24) -> ()
      n207 = control-ref of="This VI"() -> (w23:refnum<vi>)
      n208 = VISA Close(VISA resource name=w29, error in (no error)=w30) -> (error out=w28:errorcluster)
      n209 = local write "EOP"(w25) -> ()
      n210 = call <vilib>:"Simple Error Handler.vi"("error in (no error)"=w28) -> ()  [unwired: 4 in, 5 out]
    }
    frame True {
      n211 = case shown="False" w469 {
        tunnel: "LANC interface not found!" ("search string/char (-)") -> [w475 _]
        tunnel: w470 -> [w474 _]
        frame False {
          n212 = One Button Dialog(message=w475) -> ()  [unwired: 1 in, 1 out]
          n213 = VISA Close(VISA resource name=w474) -> (error out=w473:errorcluster)  [unwired: 1 in]
          n214 = call <vilib>:"Clear Errors.vi"("error in (no error)"=w473) -> ()  [unwired: 5 in, 2 out]
        }
        frame True {
        }
      }
      n215 = control-ref of="This VI"() -> (w471:refnum<vi>)
    }
  }
  n216 = invoke class="VI" method="FP.Close"(reference=w2) -> ()  [unwired: 2 in, 3 out]
  "EOP" <- FALSE ("EOP")
